vi "server.Format Client Request (String).vi"(8 "error in (no error)":errorcluster, 9 "id":string, 10 "params":refnum<class "JSON Value.lvclass">, 11 "method":string) -> (0 "error out":errorcluster, 2 "Request String":string)   [LabVIEW 2016, in "JSONRPC Server.lvclass"]
uses:
  JSONRPC Server.lvclass
  <vilib>/NI/JSON Support for LabVIEW/JSON Value/JSON Value.lvclass
  <vilib>/NI/JSON Support for LabVIEW/JSON Value/Object/Insert Value/Insert Value (String).vi
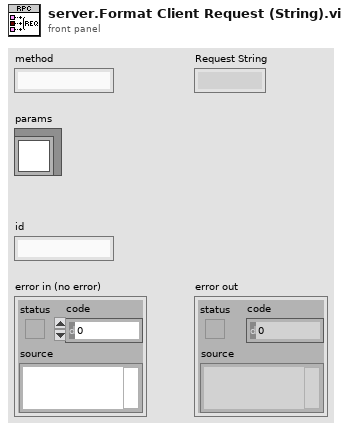
[diagram p1: front panel]
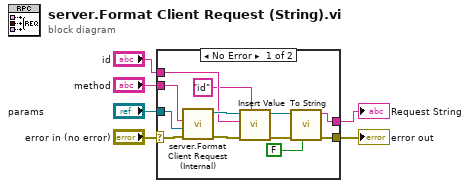
[diagram p0: block diagram]
diagram:
  n1 = case shown="No Error" "error in (no error)" {
    selector: "error in (no error)" -> [w18 w19]
    tunnel: [w17 w19] -> w5
    tunnel: "params" -> [w12 _]
    tunnel: [w16 _] -> w3
    tunnel: "method" -> [w15 _]
    tunnel: "id" -> [w10 _]
    frame No Error {
      n2 = call "server.Format Client Request (Internal).vi"("error in (no error)"=w18, "params"=w12, "method"=w15) -> ("error out"=w13:errorcluster, "JSON Value out"=w11:refnum<class "JSON Value.lvclass">)  [unwired: 7 in]
      n3 = call-poly <vilib>:"Insert Value.vi"("key"="id" ("Name"), "error in (no error)"=w13, "value"=w10, "JSON Value in"=w11) -> ("error out"=w14:errorcluster, "JSON Value out"=w8:refnum<class "JSON Value.lvclass">)  [unwired: 5 in, 1 out]
      n4 = call <vilib>:"To String.vi"("pretty print? (T)"=FALSE, "error in (no error)"=w14, "JSON Value in"=w8) -> ("error out"=w17:errorcluster, "String"=w16:string)  [unwired: 7 in]
    }
    frame Error {
    }
  }
  "error out" <- w5
  "Request String" <- w3
